vi "HW_Configure_port(s).vi"(0 "Settings cluster in":T2={"Defaults"={"Default User"=0.0, "VISA Resource Name "=""}, "Recording and saving"={"Researcher name"="", "Name prefix"="", "Data filtering"={"Filter type"=enum."Savitzky-Golay", "Length"=31, "Order"=3}, "Stop at"=0.0, "\"Stop at\" enabled"=FALSE, "Default save folder path"=path ""}, "Geometry"={"Cage diameter, mm"=0, "Starting angle MIDFIELD"=0, "Starting angle BORDER"=0, "Radius, mm CENTER"=0, "Radius, mm MIDFIELD"=0, "N segments MIDFIELD"=0, "N segments BORDER"=0, "R-gap, mm"=0.0, "Bridge swap"=FALSE, "Bridge H. offset"=0.0, "Bridge V. offset"=0.0, "Twisted neck"=FALSE, "Alt. magn. orientation"=FALSE}, "IO parameters"={"IO general config."=0, "IO 1 configuration"=0, "IO 2 configuration"=0, "IO 3 configuration"=0, "IO 4 configuration"=0, "Activate ext. RS-232"=0, "IO inversion config."=0, "Sync capability"=1}, "Stimulus presets array"=[{"Event type"=0, "Dur., s"=0.0, "Stim., s"=0.0, "TTL out N"=1, "Set/Clear"=FALSE, "Stim. has been set"=FALSE}, {"Event type"=0, "Dur., s"=0.0, "Stim., s"=0.0, "TTL out N"=1, "Set/Clear"=FALSE, "Stim. has been set"=FALSE}, {"Event type"=0, "Dur., s"=0.0, "Stim., s"=0.0, "TTL out N"=1, "Set/Clear"=FALSE, "Stim. has been set"=FALSE}, {"Event type"=0, "Dur., s"=0.0, "Stim., s"=0.0, "TTL out N"=1, "Set/Clear"=FALSE, "Stim. has been set"=FALSE}, {"Event type"=0, "Dur., s"=0.0, "Stim., s"=0.0, "TTL out N"=1, "Set/Clear"=FALSE, "Stim. has been set"=FALSE}, {"Event type"=0, "Dur., s"=0.0, "Stim., s"=0.0, "TTL out N"=1, "Set/Clear"=FALSE, "Stim. has been set"=FALSE}, {"Event type"=0, "Dur., s"=0.0, "Stim., s"=0.0, "TTL out N"=1, "Set/Clear"=FALSE, "Stim. has been set"=FALSE}, {"Event type"=0, "Dur., s"=0.0, "Stim., s"=0.0, "TTL out N"=1, "Set/Clear"=FALSE, "Stim. has been set"=FALSE}, {"Event type"=0, "Dur., s"=0.0, "Stim., s"=0.0, "TTL out N"=1, "Set/Clear"=FALSE, "Stim. has been set"=FALSE}, {"Event type"=0, "Dur., s"=0.0, "Stim., s"=0.0, "TTL out N"=1, "Set/Clear"=FALSE, "Stim. has been set"=FALSE}, {"Event type"=0, "Dur., s"=0.0, "Stim., s"=0.0, "TTL out N"=1, "Set/Clear"=FALSE, "Stim. has been set"=FALSE}, {"Event type"=0, "Dur., s"=0.0, "Stim., s"=0.0, "TTL out N"=1, "Set/Clear"=FALSE, "Stim. has been set"=FALSE}, {"Event type"=0, "Dur., s"=0.0, "Stim., s"=0.0, "TTL out N"=1, "Set/Clear"=FALSE, "Stim. has been set"=FALSE}, {"Event type"=0, "Dur., s"=0.0, "Stim., s"=0.0, "TTL out N"=1, "Set/Clear"=FALSE, "Stim. has been set"=FALSE}], "Settings loaded OK"=FALSE} {"Stimulus presets array"."Event type" items=["Stay for N seconds"]; "Stimulus presets array"."TTL out N" items=["1"=1, "2"=2, "1+2"=3]; "Recording and saving"."Data filtering"."Order" min=3 max=11 step=2; "Recording and saving"."Data filtering"."Length" min=5 max=301 step=2; "Geometry"."Cage diameter, mm" scale=0.0..340.0}, 1 "error in (no error)":errorcluster) -> (2 "Settings cluster out":T2={"Defaults"={"Default User"=0.0, "VISA Resource Name "=""}, "Recording and saving"={"Researcher name"="", "Name prefix"="", "Data filtering"={"Filter type"=enum."Savitzky-Golay", "Length"=31, "Order"=3}, "Stop at"=0.0, "\"Stop at\" enabled"=FALSE, "Default save folder path"=path ""}, "Geometry"={"Cage diameter, mm"=0, "Starting angle MIDFIELD"=0, "Starting angle BORDER"=0, "Radius, mm CENTER"=0, "Radius, mm MIDFIELD"=0, "N segments MIDFIELD"=0, "N segments BORDER"=0, "R-gap, mm"=0.0, "Bridge swap"=FALSE, "Bridge H. offset"=0.0, "Bridge V. offset"=0.0, "Twisted neck"=FALSE, "Alt. magn. orientation"=FALSE}, "IO parameters"={"IO general config."=0, "IO 1 configuration"=0, "IO 2 configuration"=0, "IO 3 configuration"=0, "IO 4 configuration"=0, "Activate ext. RS-232"=0, "IO inversion config."=0, "Sync capability"=1}, "Stimulus presets array"=[{"Event type"=0, "Dur., s"=0.0, "Stim., s"=0.0, "TTL out N"=1, "Set/Clear"=FALSE, "Stim. has been set"=FALSE}, {"Event type"=0, "Dur., s"=0.0, "Stim., s"=0.0, "TTL out N"=1, "Set/Clear"=FALSE, "Stim. has been set"=FALSE}, {"Event type"=0, "Dur., s"=0.0, "Stim., s"=0.0, "TTL out N"=1, "Set/Clear"=FALSE, "Stim. has been set"=FALSE}, {"Event type"=0, "Dur., s"=0.0, "Stim., s"=0.0, "TTL out N"=1, "Set/Clear"=FALSE, "Stim. has been set"=FALSE}, {"Event type"=0, "Dur., s"=0.0, "Stim., s"=0.0, "TTL out N"=1, "Set/Clear"=FALSE, "Stim. has been set"=FALSE}, {"Event type"=0, "Dur., s"=0.0, "Stim., s"=0.0, "TTL out N"=1, "Set/Clear"=FALSE, "Stim. has been set"=FALSE}, {"Event type"=0, "Dur., s"=0.0, "Stim., s"=0.0, "TTL out N"=1, "Set/Clear"=FALSE, "Stim. has been set"=FALSE}, {"Event type"=0, "Dur., s"=0.0, "Stim., s"=0.0, "TTL out N"=1, "Set/Clear"=FALSE, "Stim. has been set"=FALSE}, {"Event type"=0, "Dur., s"=0.0, "Stim., s"=0.0, "TTL out N"=1, "Set/Clear"=FALSE, "Stim. has been set"=FALSE}, {"Event type"=0, "Dur., s"=0.0, "Stim., s"=0.0, "TTL out N"=1, "Set/Clear"=FALSE, "Stim. has been set"=FALSE}, {"Event type"=0, "Dur., s"=0.0, "Stim., s"=0.0, "TTL out N"=1, "Set/Clear"=FALSE, "Stim. has been set"=FALSE}, {"Event type"=0, "Dur., s"=0.0, "Stim., s"=0.0, "TTL out N"=1, "Set/Clear"=FALSE, "Stim. has been set"=FALSE}, {"Event type"=0, "Dur., s"=0.0, "Stim., s"=0.0, "TTL out N"=1, "Set/Clear"=FALSE, "Stim. has been set"=FALSE}, {"Event type"=0, "Dur., s"=0.0, "Stim., s"=0.0, "TTL out N"=1, "Set/Clear"=FALSE, "Stim. has been set"=FALSE}], "Settings loaded OK"=FALSE} {"Stimulus presets array"."Event type" items=["Stay for N seconds"]; "Stimulus presets array"."TTL out N" items=["1"=1, "2"=2, "1+2"=3]; "Recording and saving"."Data filtering"."Order" min=3 max=11 step=2; "Recording and saving"."Data filtering"."Length" min=5 max=301 step=2; "Geometry"."Cage diameter, mm" scale=0.0..340.0}, 3 "Data updated":bool, 4 "error out":errorcluster)   [LabVIEW 2018]
uses:
  Controls/CTL_Undo_button.ctl
  Controls/CTL_Settings_cluster.ctl
  Controls/CTL_Filter_selector.ctl
  Controls/CTL_Segmented_plot_parameters.ctl
  Controls/CTL_IO_params_cluster.ctl
  Controls/CTL_Single_stimulus_setting.ctl
  Controls/CTL_VISA_port_Descr.-Name.ctl
  <vilib>/Utility/miscctls.llb/LVPointTypeDef.ctl
panel:
  out "Current port":string
  in  "COM-ports":i32(listbox)
  out "Detected COM ports":T1[](array[typedef])
  out "Previous parameters":cluster{"VISA resourse name":string}
  in  "Check HW":bool
  in  "Undo":T7
  in  "Save Config":bool
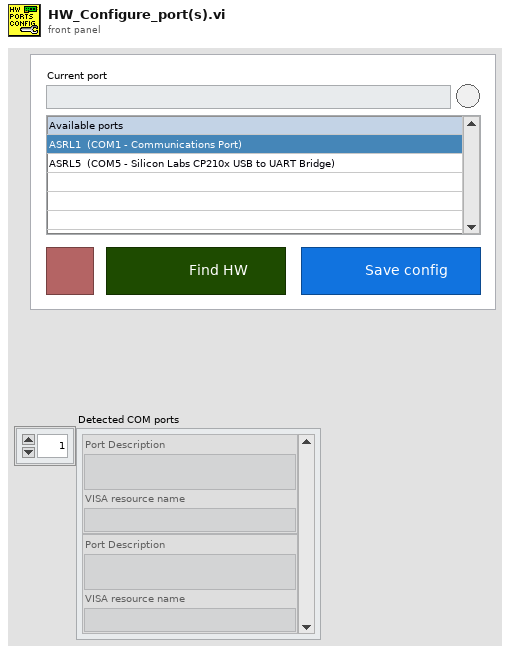
[diagram p1: front panel]
types:
  T1 = typedef "CTL_VISA_port_Descr.-Name.ctl" = cluster{"Port Description":string, "VISA resource name":string}
  T2 = typedef "CTL_Settings_cluster.ctl" = cluster{"Defaults":cluster{"Default User":dbl, "VISA Resource Name ":string}, "Recording and saving":cluster{"Researcher name":string, "Name prefix":string, "Data filtering":T3, "Stop at":dbl, "\"Stop at\" enabled":bool, "Default save folder path":path}, "Geometry":T4, "IO parameters":T5, "Stimulus presets array":T6[], "Settings loaded OK":bool}
  T3 = typedef "CTL_Filter_selector.ctl" = cluster{"Filter type":enum16{"None", "Savitzky-Golay"}, "Length":i32, "Order":i32}
  T4 = typedef "CTL_Segmented_plot_parameters.ctl" = cluster{"Cage diameter, mm":u16, "Starting angle MIDFIELD":i16, "Starting angle BORDER":i16, "Radius, mm CENTER":u16, "Radius, mm MIDFIELD":u16, "N segments MIDFIELD":u8, "N segments BORDER":u8, "R-gap, mm":sgl, "Bridge swap":bool, "Bridge H. offset":sgl, "Bridge V. offset":sgl, "Twisted neck":bool, "Alt. magn. orientation":bool}
  T5 = typedef "CTL_IO_params_cluster.ctl" = cluster{"IO general config.":u16, "IO 1 configuration":u16, "IO 2 configuration":u16, "IO 3 configuration":u16, "IO 4 configuration":u16, "Activate ext. RS-232":u16, "IO inversion config.":u16, "Sync capability":u8}
  T6 = typedef "CTL_Single_stimulus_setting.ctl" = cluster{"Event type":u16, "Dur., s":sgl, "Stim., s":sgl, "TTL out N":u16, "Set/Clear":bool, "Stim. has been set":bool}
  T7 = typedef "CTL_Undo_button.ctl" = bool
  T8 = typedef "LVPointTypeDef.ctl" = cluster{"Horizontal":i16, "Vertical":i16}
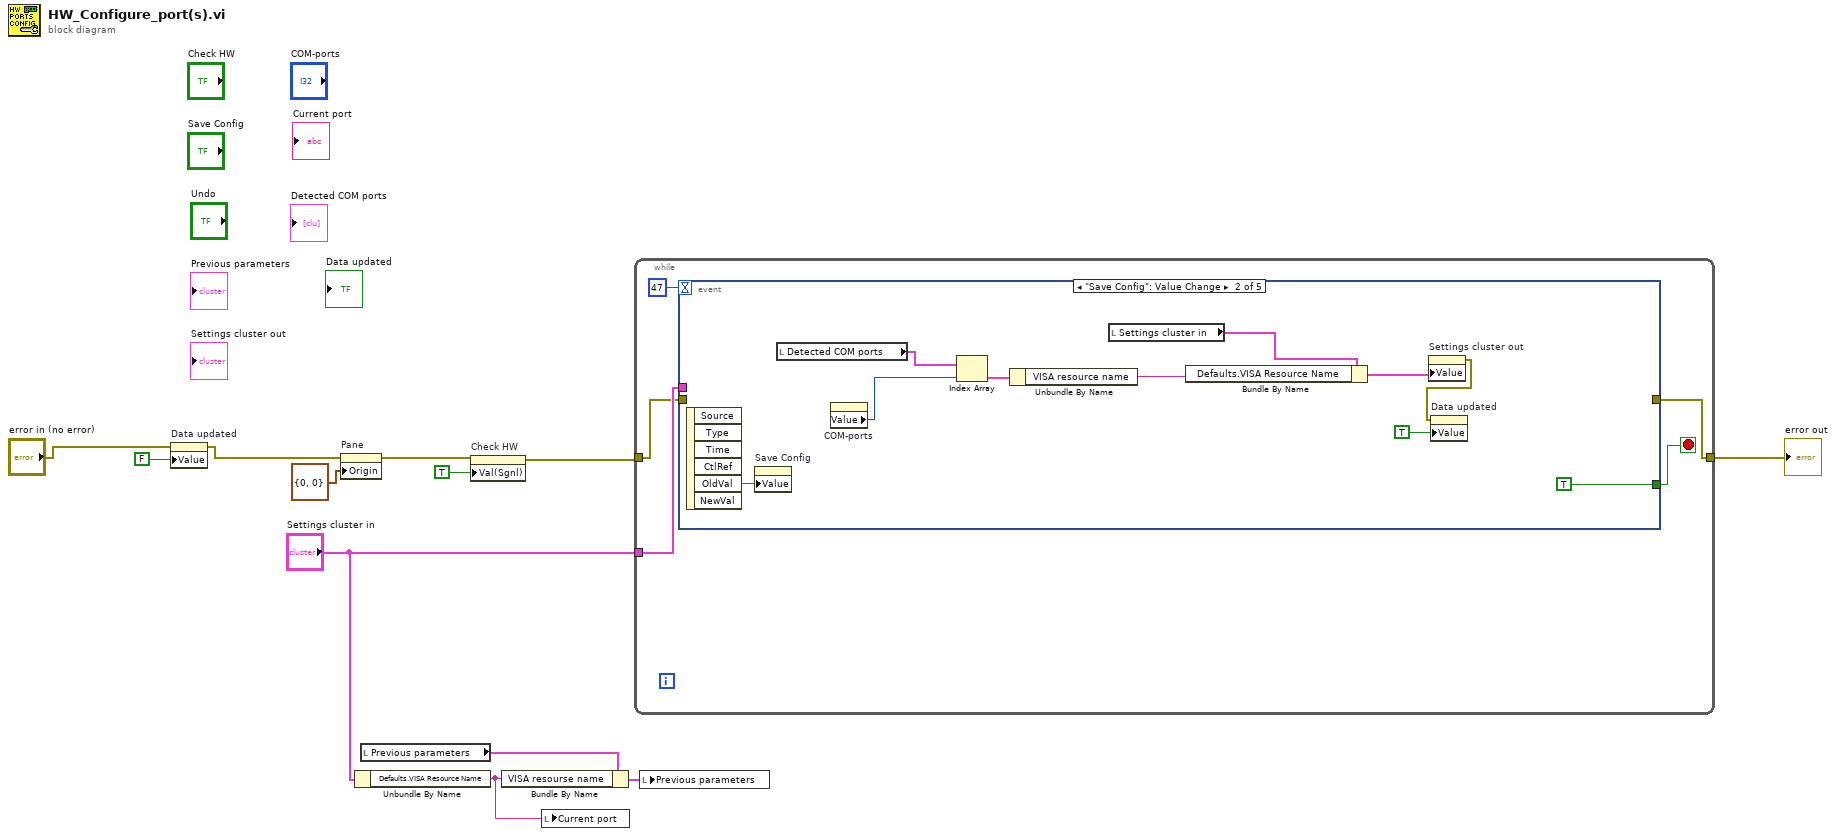
[diagram p0: block diagram]
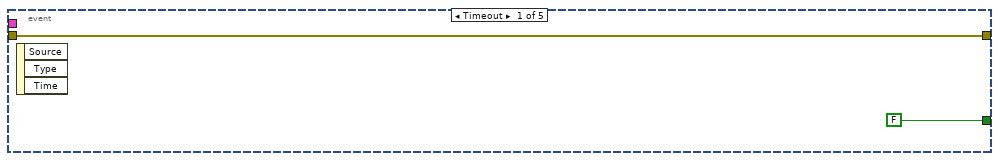
[diagram p2: hidden frame]
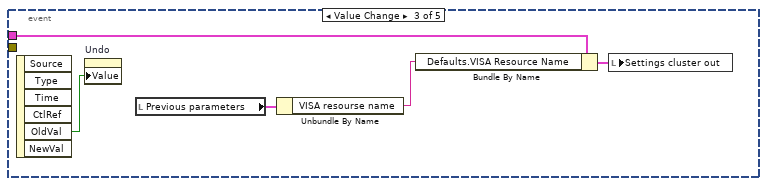
[diagram p3: hidden frame]
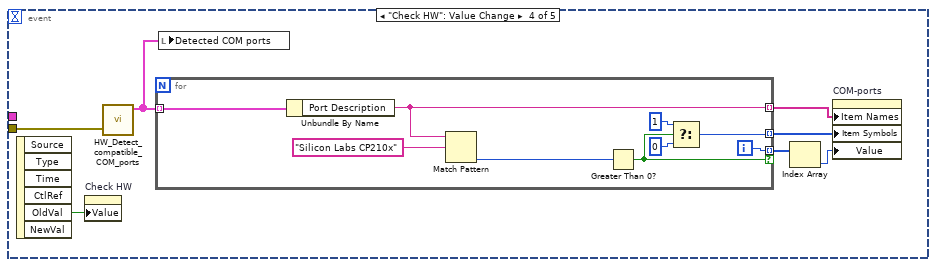
[diagram p4: hidden frame]
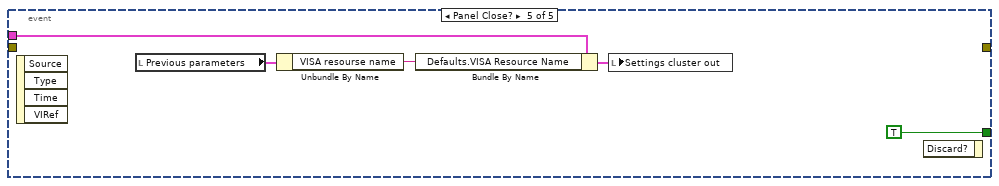
[diagram p5: hidden frame]
diagram:
  n1 = property on="Data updated" class="Bool (strict)"(error in="error in (no error)", "Value"=FALSE ("Data updated")) -> (error out=w2:errorcluster)  [unwired: 1 in, 1 out]
  n2 = property on="Pane" class="Pane"(error in=w2, "Origin"=T8 {"Horizontal"=0, "Vertical"=0}) -> (error out=w7:errorcluster)  [unwired: 1 in, 1 out]
  n3 = Unbundle By Name("Settings cluster in") -> ("Defaults.VISA Resource Name"=w4:string)
  n4 = local read "Previous parameters"() -> (w9:cluster{"VISA resourse name":string})
  n5 = property on="Check HW" class="Bool (strict)"(error in=w7, "Val(Sgnl)"=TRUE ("Value (Signaling)")) -> (error out=w6:errorcluster)  [unwired: 1 in, 1 out]
  n6 = Bundle By Name(cluster=w9, "VISA resourse name"=w4) -> (w8:cluster{"VISA resourse name":string})
  n7 = local write "Current port"(w4) -> ()
  n8 = while {
    tunnel: "Settings cluster in" -> [w15]
    tunnel: w6 -> [w13]
    tunnel: [w14] -> w11
    stop <- w16 stop-if-true
    n9 = event shown="[1] \"Save Config\": Value Change" {
      selector: _ -> [_ _ _ _ _]
      dyn-events: _ -> [_ _ _ _ _]
      timeout: 47 -> [_ _ _ _ _]
      tunnel: [FALSE TRUE _ _ TRUE] -> w16
      tunnel: w15 -> [_ _ w33 _ w54]
      tunnel: [w18 _ _ _ _] -> w14
      tunnel: w13 -> [w18 _ _ w40 _]
      event Timeout {
        n10 = event-data() -> ()  [unwired: 1 in, 3 out]
      }
      event "Save Config": Value Change {
        n11 = event-data() -> ("OldVal"=w28:bool)  [unwired: 1 in, 5 out]
        n12 = property on="Save Config" class="Bool (strict)"("Value"=w28) -> ()  [unwired: 2 in, 2 out]
        n13 = local read "Detected COM ports"() -> (w27:T1[])
        n14 = property on="COM-ports" class="LstBox (strict)"() -> ("Value"=w26:i32)  [unwired: 2 in, 2 out]
        n15 = Index Array(array=w27, index=w26) -> (element=w25:T1)
        n16 = Unbundle By Name(w25) -> ("VISA resource name"=w24:string)
        n17 = local read "Settings cluster in"() -> (w20:T2)
        n18 = Bundle By Name(cluster=w20, "Defaults.VISA Resource Name"=w24) -> (w23:T2)
        n19 = property on="Settings cluster out" class="Clust (strict)"("Value"=w23) -> (error out=w21:errorcluster)  [unwired: 2 in, 1 out]
        n20 = property on="Data updated" class="Bool (strict)"(error in=w21, "Value"=TRUE ("Data updated")) -> ()  [unwired: 1 in, 2 out]
      }
      event Value Change {
        n21 = event-data() -> ("OldVal"=w34:T7)  [unwired: 1 in, 5 out]
        n22 = property on="Undo" class="Bool (strict)"("Value"=w34) -> ()  [unwired: 2 in, 2 out]
        n23 = local read "Previous parameters"() -> (w32:cluster{"VISA resourse name":string})
        n24 = Unbundle By Name(w32) -> ("VISA resourse name"=w31:string)
        n25 = Bundle By Name(cluster=w33, "Defaults.VISA Resource Name"=w31) -> (w30:T2)
        n26 = local write "Settings cluster out"(w30) -> ()
      }
      event "Check HW": Value Change {
        n27 = event-data() -> ("OldVal"=w41:bool)  [unwired: 1 in, 5 out]
        n28 = property on="Check HW" class="Bool (strict)"("Value"=w41) -> ()  [unwired: 2 in, 2 out]
        n29 = call "HW_Detect_compatible_COM_ports.vi"("Error In"=w40) -> ("Detected COM ports"=w35:T1[])  [unwired: 1 in, 3 out]
        n30 = for {
          tunnel: w35 -> [w50] mode=indexing
          tunnel: [w49] -> w39 mode=indexing
          tunnel: [w46] -> w37 mode=indexing if=w45
          tunnel: [w44] -> w38 mode=indexing
          i -> [w46]
          n31 = Unbundle By Name(w50) -> ("Port Description"=w49:string)
          n32 = Match Pattern(string=w49, regular expression="Silicon Labs CP210x") -> (offset past match=w47:i32)  [unwired: 1 in, 3 out]
          n33 = Greater Than 0?(x=w47) -> (x > 0?=w45:bool)
          n34 = Select(t=1, s=w45, f=0) -> (s? t:f=w44:i32)
        }
        n35 = local write "Detected COM ports"(w35) -> ()
        n36 = Index Array(array=w37) -> (element=w36:i32)  [unwired: 1 in]
        n37 = property on="COM-ports" class="LstBox (strict)"("Item Names"=w39, "Item Symbols"=w38, "Value"=w36) -> ()  [unwired: 2 in, 2 out]
      }
      event Panel Close? {
        n38 = event-data() -> ()  [unwired: 1 in, 4 out]
        n39 = local read "Previous parameters"() -> (w51:cluster{"VISA resourse name":string})
        n40 = Unbundle By Name(w51) -> ("VISA resourse name"=w53:string)
        n41 = Bundle By Name(cluster=w54, "Defaults.VISA Resource Name"=w53) -> (w52:T2)
        n42 = local write "Settings cluster out"(w52) -> ()
        n43 = event-data() -> ()  [unwired: 2 in, 1 out]
      }
    }
  }
  "error out" <- w11
  n44 = local write "Previous parameters"(w8) -> ()
